vi "Flywheel Tach.vi"() -> ()   [LabVIEW 2013]
uses:
  Robot Global Data.vi
panel:
  out "RPM Top":dbl
  out "RPM Bottom":dbl
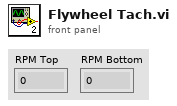
[diagram p1: front panel]
types:
  T1 = typedef "WPI_CounterDevRef.ctl" = cluster{"DevStatus":errorcluster, "CntIndex":T2}
  T2 = typedef "FPGA_CounterCtrSystemIndex.ctl" = enum8{"Ctr 0", "Ctr 1", "Ctr 2", "Ctr 3", "Ctr 4", "Ctr 5", "Ctr 6", "Ctr 7", "Invalid"}
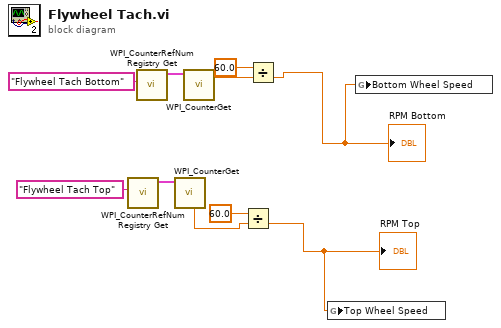
[diagram p0: block diagram]
diagram:
  n1 = call <vilib>:"WPI_CounterRefNum Registry Get.vi"("refnum name"="Flywheel Tach Top") -> ("CounterDevRef"=w7:T1)  [unwired: 9 in, 1 out]
  n2 = call <vilib>:"WPI_CounterRefNum Registry Get.vi"("refnum name"="Flywheel Tach Bottom") -> ("CounterDevRef"=w9:T1)  [unwired: 9 in, 1 out]
  n3 = call <vilib>:"WPI_CounterGet.vi"("CounterDevRef in"=w7) -> ("Period (sec)"=w5:dbl)  [unwired: 5 in, 5 out]
  n4 = call <vilib>:"WPI_CounterGet.vi"("CounterDevRef in"=w9) -> ("Period (sec)"=w6:dbl)  [unwired: 5 in, 5 out]
  n5 = Divide(x=60.0, y=w5) -> (x/y=w1:dbl)
  "RPM Top" <- w1
  n6 = Divide(x=60.0, y=w6) -> (x/y=w2:dbl)
  "RPM Bottom" <- w2
  n7 = global write "Robot Global Data.vi" "Top Wheel Speed"(w1) -> ()
  n8 = global write "Robot Global Data.vi" "Bottom Wheel Speed"(w2) -> ()
